vi "addToScanLog.vi"(0 "Model in":refnum<class "Model.lvclass">, 5 "Control Value":dbl, 7 "Measured Force":dbl[unit], 9 "Measured Pressure":dbl[unit], 11 "error in (no error)":errorcluster) -> (4 "Model out":refnum<class "Model.lvclass">, 15 "error out":errorcluster)   [LabVIEW 2015, in "Model.lvclass"]
uses:
  Model.lvclass
  Model.lvclass/Model.ctl
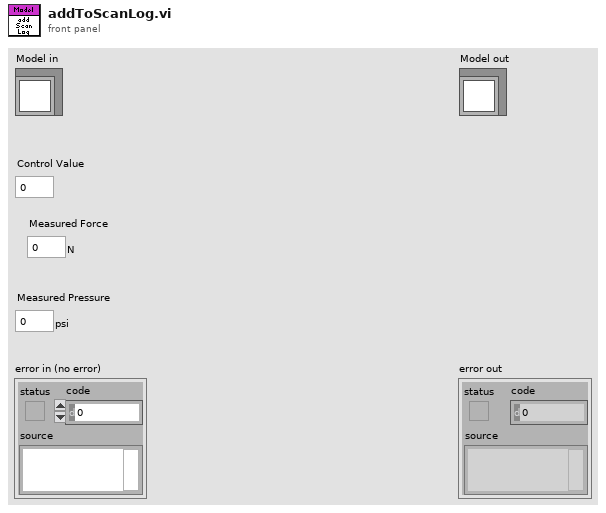
[diagram p1: front panel]
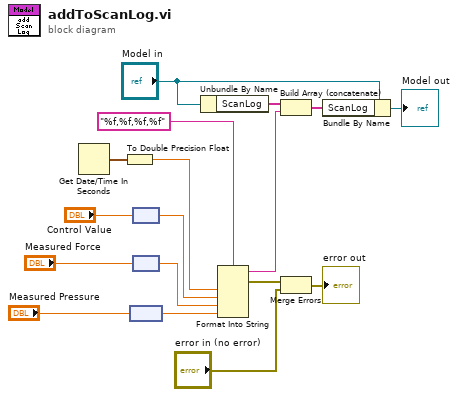
[diagram p0: block diagram]
diagram:
  n1 = Get Date/Time In Seconds() -> (seconds since 1Jan1904=w3:timestamp)
  n2 = To Double Precision Float(number=w3) -> (double precision float=w1:dbl)
  n3 = node("Measured Pressure") -> (w4:dbl)
  n4 = node("Control Value") -> (w2:dbl[unit])
  n5 = node("Measured Force") -> (w6:dbl)
  n6 = Unbundle By Name("Model in") -> ("ScanLog"=w17:string[])
  n7 = Format Into String(format string="%f,%f,%f,%f", w1, w2, w6, w4) -> (resulting string=w13:string, error out=w11:errorcluster)  [unwired: 2 in]
  n8 = Build Array (concatenate)(w17, w13) -> (w12:string[])
  n9 = Merge Errors(w11, "error in (no error)") -> (→"error out":errorcluster)
  n10 = Bundle By Name(cluster="Model in", "ScanLog"=w12) -> (→"Model out":refnum<class "Model.lvclass">)
